vi "Write RFx.vi"(8 "error in (no error)":errorcluster, 10 "RFx":bool[](array[boolean])=[TRUE, TRUE, TRUE, TRUE], 11 "WS5100 in":refnum<class "WS5100.lvclass">) -> (0 "error out":errorcluster, 3 "WS5100 out":refnum<class "WS5100.lvclass">)   [LabVIEW 2020, in "WS5100.lvclass"]
uses:
  WS5100.lvclass
  WS5100.lvclass/WS5100.ctl
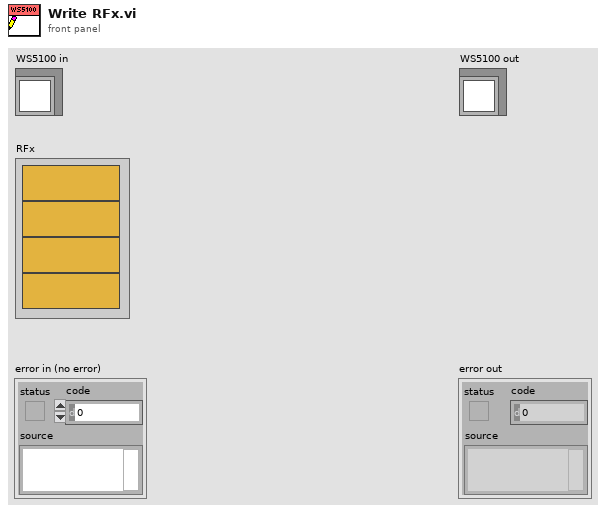
[diagram p1: front panel]
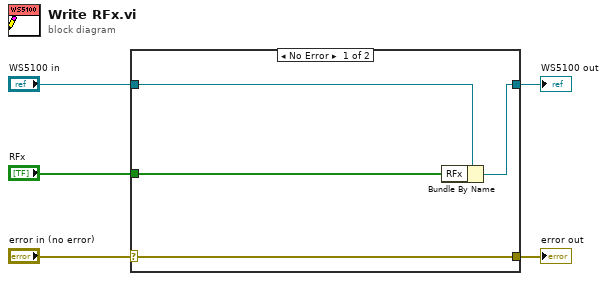
[diagram p0: block diagram]
diagram:
  n1 = case shown="No Error" "error in (no error)" {
    selector: "error in (no error)" -> [w9 w10]
    tunnel: [w9 w10] -> w4
    tunnel: [w7 w11] -> w2
    tunnel: "WS5100 in" -> [w8 w11]
    tunnel: "RFx" -> [w6 _]
    frame No Error {
      n2 = Bundle By Name(cluster=w8, "RFx"=w6) -> (w7:refnum<class "WS5100.lvclass">)
    }
    frame Error {
    }
  }
  "error out" <- w4
  "WS5100 out" <- w2
